vi "Read Until Match.vi"(6 "Regular Expression?":bool, 8 "error in (no error)":errorcluster, 9 "Timeout S (0)":dbl, 10 "Match String":string, 11 "DeployResource in":refnum<class "DeployResource.lvclass">) -> (0 "error out":errorcluster, 1 "Found?":bool, 2 "Data":string, 3 "DeployResource out":refnum<class "DeployResource.lvclass">)   [LabVIEW 2020, in "PicoG-Core.lvlib" / "DeployResource.lvclass"]
uses:
  DeployResource.lvclass
  <vilib>/regexp/Match Regular Expression.xnode
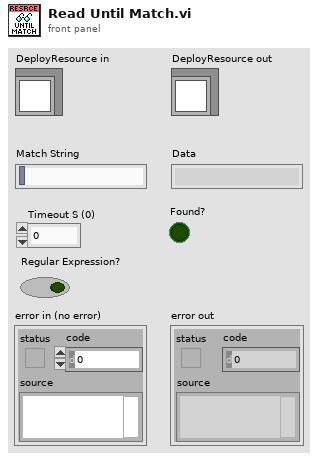
[diagram p1: front panel]
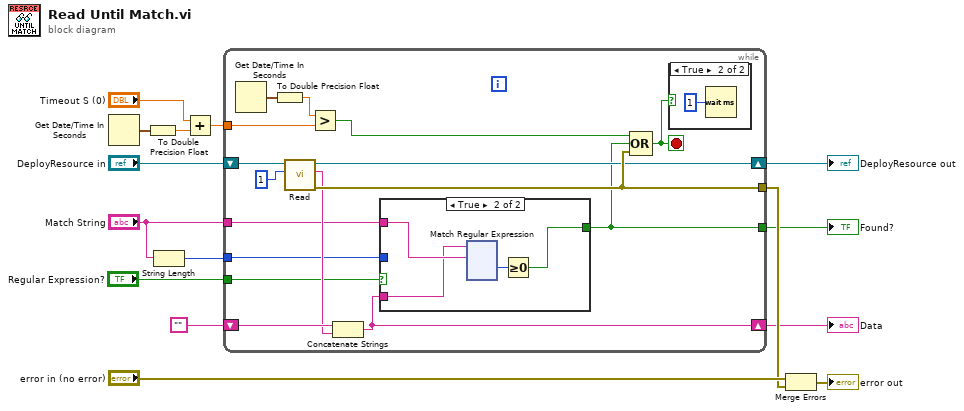
[diagram p0: block diagram]
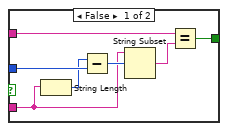
[diagram p2: hidden frame]
diagram:
  n1 = Get Date/Time In Seconds() -> (seconds since 1Jan1904=w11:timestamp)
  n2 = To Double Precision Float(number=w11) -> (double precision float=w10:dbl)
  n3 = String Length(string="Match String") -> (length=w14:i32)
  n4 = Add(x="Timeout S (0)", y=w10) -> (x+y=w8:dbl)
  n5 = while {
    shift-right: [w29] -> w12
    shift-left: "DeployResource in" -> [w30]
    tunnel: w8 -> [w27]
    tunnel: "Match String" -> [w20]
    shift-right: [w17] -> w2
    shift-left: "" -> [w23]
    tunnel: w14 -> [w21]
    tunnel: [w31] -> w5
    tunnel: [w18] -> w4
    tunnel: "Regular Expression?" -> [w16]
    stop <- w24 stop-if-true
    n6 = Get Date/Time In Seconds() -> (seconds since 1Jan1904=w28:timestamp)
    n7 = To Double Precision Float(number=w28) -> (double precision float=w26:dbl)
    n8 = call-dynamic "Read.vi"("Bytes to Read (0)"=1, "DeployResource in"=w30) -> ("error out"=w31:errorcluster, "Data"=w22:string, "DeployResource out"=w29:refnum<class "DeployResource.lvclass">)  [unwired: 6 in, 1 out]
    n9 = Greater?(x=w26, y=w27) -> (0:w25:bool)
    n10 = Concatenate Strings(w23, w22) -> (w17:string)
    n11 = case shown="True" w16 {
      tunnel: w21 -> [w38 _]
      tunnel: w20 -> [w36 w42]
      tunnel: [w35 w39] -> w18
      tunnel: w17 -> [w33 w41]
      frame False {
        n12 = String Length(string=w33) -> (length=w37:i32)
        n13 = Subtract(x=w37, y=w38) -> (x-y=w34:i32)
        n14 = String Subset(string=w33, offset (0)=w34) -> (substring=w32:string)  [unwired: 1 in]
        n15 = Equal?(x=w36, y=w32) -> (x = y?=w35:bool)
      }
      frame True {
        n16 = xnode "Match Regular Expression"("input string"=w41, "regular expression"=w42) -> ("offset past match"=w40:i32)  [unwired: 4 in, 4 out]
        n17 = Greater Or Equal To 0?(x=w40) -> (x >= 0?=w39:bool)
      }
    }
    n18 = Compound Arithmetic op=OR(w25, w18, w31) -> (w24:bool)
    n19 = case shown="True" w24 {
      frame False {
      }
      frame True {
        n20 = Wait (ms)(milliseconds to wait=u32 1) -> ()  [unwired: 1 out]
      }
    }
  }
  "DeployResource out" <- w12
  "Data" <- w2
  "Found?" <- w4
  n21 = Merge Errors("error in (no error)", w5) -> (→"error out":errorcluster)
